vi "xy_graph.vi"() -> ()   [LabVIEW 2022 SP3]
panel:
  out "XY Graph":cluster{dbl[], dbl[]}(graph)
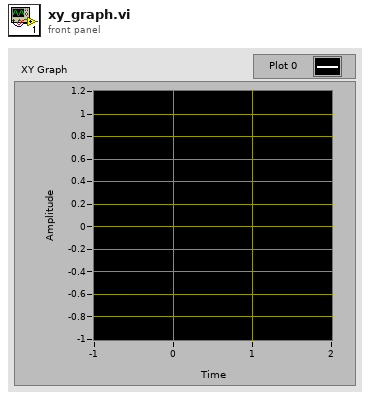
[diagram p1: front panel]
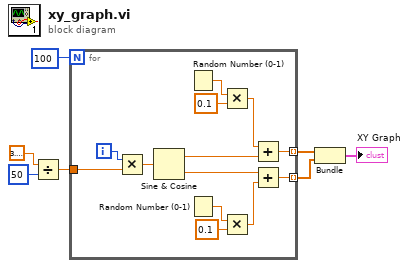
[diagram p0: block diagram]
diagram:
  n1 = Divide(x=3.141592653589793, y=50) -> (x/y=w1:dbl)
  n2 = for {
    N: 100 -> [_]
    tunnel: [w17] -> w6 mode=indexing
    tunnel: [w19] -> w5 mode=indexing
    tunnel: w1 -> [w15]
    i -> [w16]
    n3 = Multiply(x=w16, y=w15) -> (x*y=w14:dbl)
    n4 = Sine & Cosine(0:w14) -> (1:w18:dbl, 2:w20:dbl)
    n5 = Random Number (0-1)() -> (number: 0 to 1=w13:dbl)
    n6 = Random Number (0-1)() -> (number: 0 to 1=w9:dbl)
    n7 = Multiply(x=w13, y=0.1) -> (x*y=w12:dbl)
    n8 = Multiply(x=w9, y=0.1) -> (x*y=w8:dbl)
    n9 = Add(x=w12, y=w18) -> (x+y=w17:dbl)
    n10 = Add(x=w20, y=w8) -> (x+y=w19:dbl)
  }
  n11 = Bundle(w6, w5) -> (→"XY Graph":cluster{dbl[], dbl[]})  [unwired: 1 in]
